vi "S7_Open.vi"(0 "IP 地址":string, 5 "PLC 系列":u8(ring) items=["S7-1200.200.200SMART"=0, "S7-300"=2, "S7-400"=3], 7 "超时（MS）":i32, 11 "error in":errorcluster) -> (4 "TCP":refnum<k5>, 6 "连接":bool, 15 "error out":errorcluster)   [LabVIEW 2014]
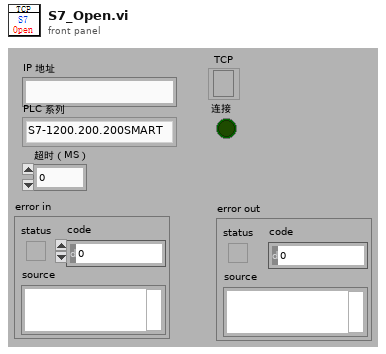
[diagram p1: front panel]
types:
  T1 = enum16{"Standard", "Buffered", "CRLF", "Immediate"}
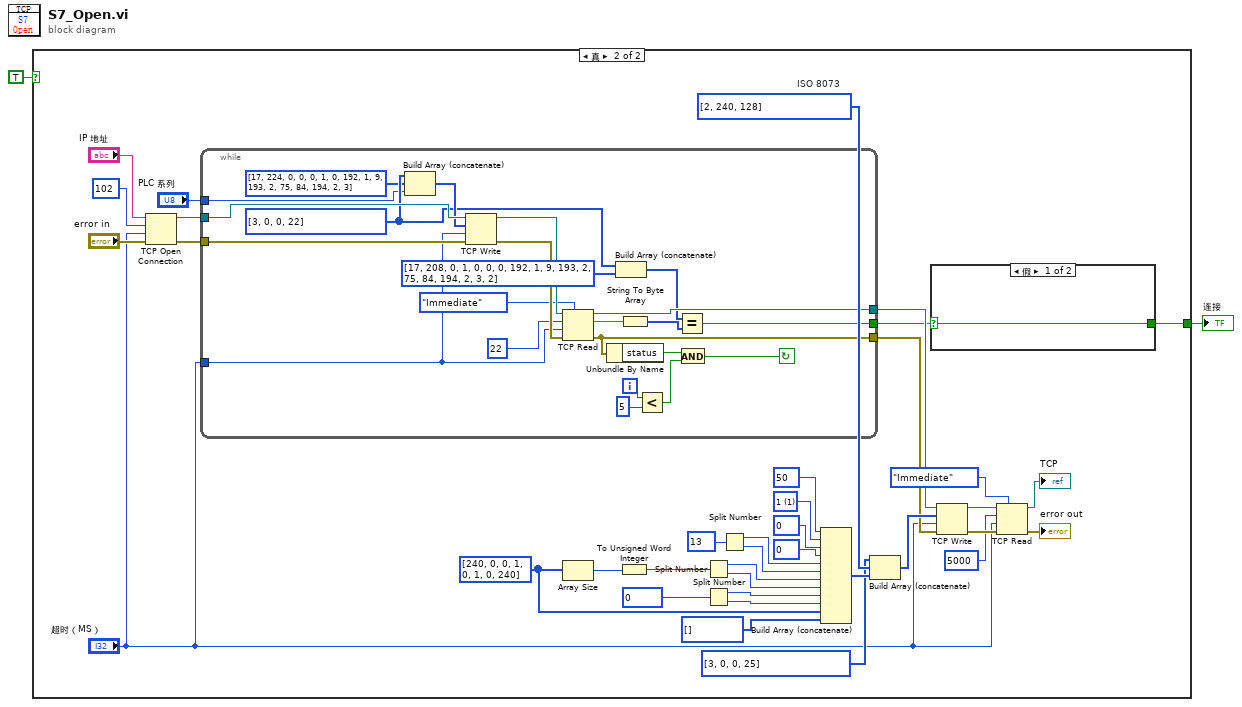
[diagram p0: block diagram]
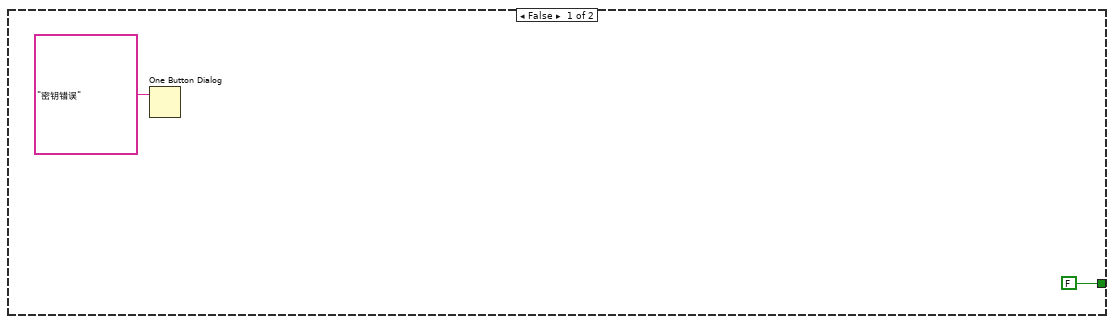
[diagram p2: hidden frame]
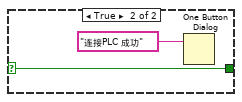
[diagram p3: hidden frame]
diagram:
  n1 = case shown="真" TRUE {
    tunnel: [FALSE w6] -> w2
    frame False {
      n2 = One Button Dialog(message="密钥错误" ("消息")) -> ()  [unwired: 2 out]
    }
    frame True {
      w24 = u8 1 items=["1"=1, "2"=2, "3"=3, "7"=7]
      w13 = u8[] [240, 0, 0, 1, 0, 1, 0, 240] ("Exchange Parameters")
      w11 = u8[] [2, 240, 128]  # ISO 8073
      n3 = TCP Open Connection(address="IP 地址", remote port or service name=u16 102, timeout ms (60000)="超时（MS）", error in (no error)="error in") -> (connection ID=w32:refnum<k5>, error out=w31:errorcluster)  [unwired: 1 out]
      n4 = while {
        tunnel: w32 -> [w61]
        tunnel: w31 -> [w60]
        tunnel: [w57] -> w30
        tunnel: [w67] -> w7
        tunnel: "PLC 系列" -> [w46]
        tunnel: [w47] -> w28
        tunnel: "超时（MS）" -> [w45]
        i -> [w65]
        stop <- w66 continue-if-true
        w51 = u8[] [3, 0, 0, 22] ("TPKT")
        n5 = Build Array (concatenate)(w51, u8[] [17, 224, 0, 0, 0, 1, 0, 192, 1, 9, 193, 2, 75, 84, 194, 2, 3] ("Connect to Adapter"), w46) -> (w53:u8[])
        n6 = TCP Write(connection ID=w61, data in=w53, error in (no error)=w60, 9:w45) -> (connection ID out=w59:refnum<k5>, error out=w58:errorcluster)  [unwired: 1 out]
        n7 = TCP Read(connection ID=w59, bytes to read=22, error in (no error)=w58, 7:T1."Immediate" ("mode (standard)"), 9:w45) -> (connection ID out=w57:refnum<k5>, data out=w54:string, error out=w47:errorcluster)
        n8 = Unbundle By Name(w47) -> ("status"=w62:bool)
        n9 = Build Array (concatenate)(w51, u8[] [17, 208, 0, 1, 0, 0, 0, 192, 1, 9, 193, 2, 75, 84, 194, 2, 3, 2] ("Connected to Adapter")) -> (w49:u8[])
        n10 = String To Byte Array(string=w54) -> (unsigned byte array=w50:u8[])
        n11 = Less?(x=w65, y=5) -> (x < y?=w63:bool)
        n12 = Equal?(x=w49, y=w50) -> (x = y?=w67:bool)
        n13 = And(x=w62, y=w63) -> (x .and. y?=w66:bool)
      }
      n14 = Array Size(array=w13) -> (size(s)=w15:i32)
      n15 = To Unsigned Word Integer(number=w15) -> (unsigned 16bit integer=w14:u16)
      n16 = Split Number(x=w14) -> (hi(x)=w27:u8, lo(x)=w22:u8)
      n17 = Split Number(x=u16 0 ("DLE")) -> (hi(x)=w21:u8, lo(x)=w20:u8)
      n18 = Split Number(x=u16 13 ("DLE")) -> (hi(x)=w17:u8, lo(x)=w16:u8)
      n19 = Build Array (concatenate)(u8 50 ("DLE"), w24, u8 0 ("DLE"), u8 0 ("DLE"), w17, w16, w27, w22, w21, w20, w13, u8[] []) -> (w10:u8[])
      n20 = Build Array (concatenate)(u8[] [3, 0, 0, 25] ("TPKT"), w11, w10) -> (w29:u8[])
      n21 = case shown="假" w7 {
        selector: w7 -> [w42 w44]
        tunnel: [w42 w44] -> w6
        frame False {
        }
        frame True {
          n22 = One Button Dialog(message="连接PLC 成功" ("消息")) -> ()  [unwired: 2 out]
        }
      }
      n23 = TCP Write(connection ID=w30, data in=w29, error in (no error)=w28, 9:"超时（MS）") -> (connection ID out=w38:refnum<k5>, error out=w37:errorcluster)  [unwired: 1 out]
      n24 = TCP Read(connection ID=w38, bytes to read=5000, error in (no error)=w37, 7:T1."Immediate" ("mode (standard)"), 9:"超时（MS）") -> (connection ID out=→"TCP":refnum<k5>, error out=→"error out":errorcluster)  [unwired: 1 out]
    }
  }
  "连接" <- w2
